vi "RFFE_Readback All Registers.vi"(8 "error out":errorcluster, 10 "RB All Regs":bool=TRUE, 11 "VISA IN":refnum<visa-resource-name>) -> (0 "error out 2":errorcluster, 2 "ALL Regs RB":string[](array[string]), 3 "VISA OUT":refnum<visa-resource-name>)   [LabVIEW 2017]
panel:
  out "Status":string="Idle....."
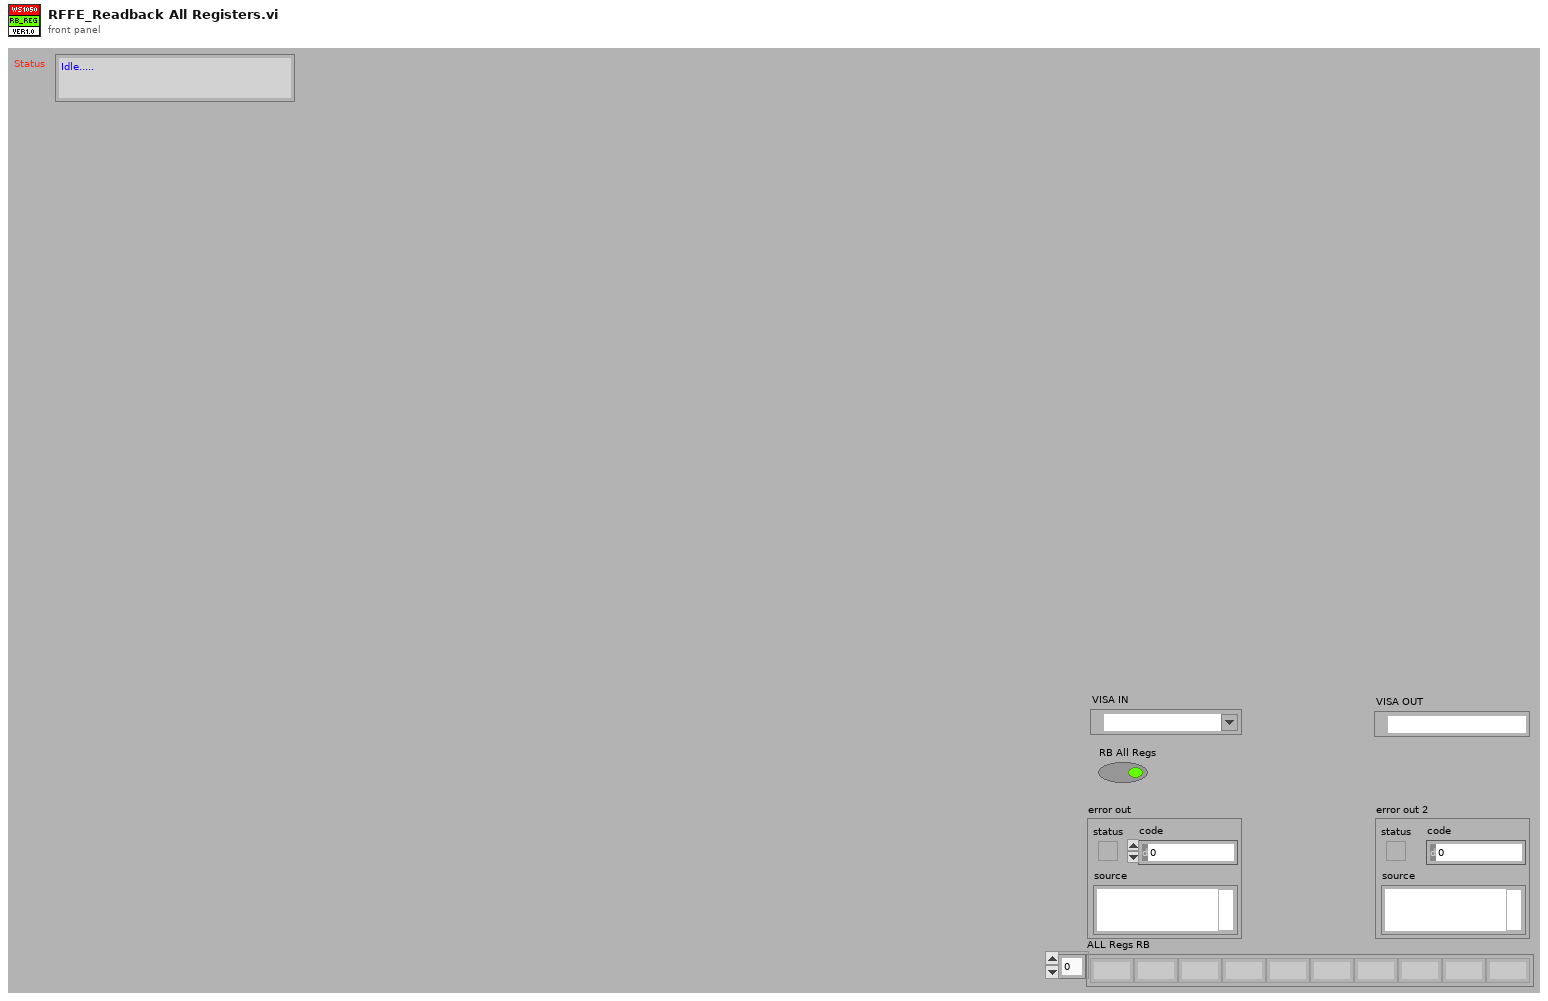
[diagram p1: front panel]
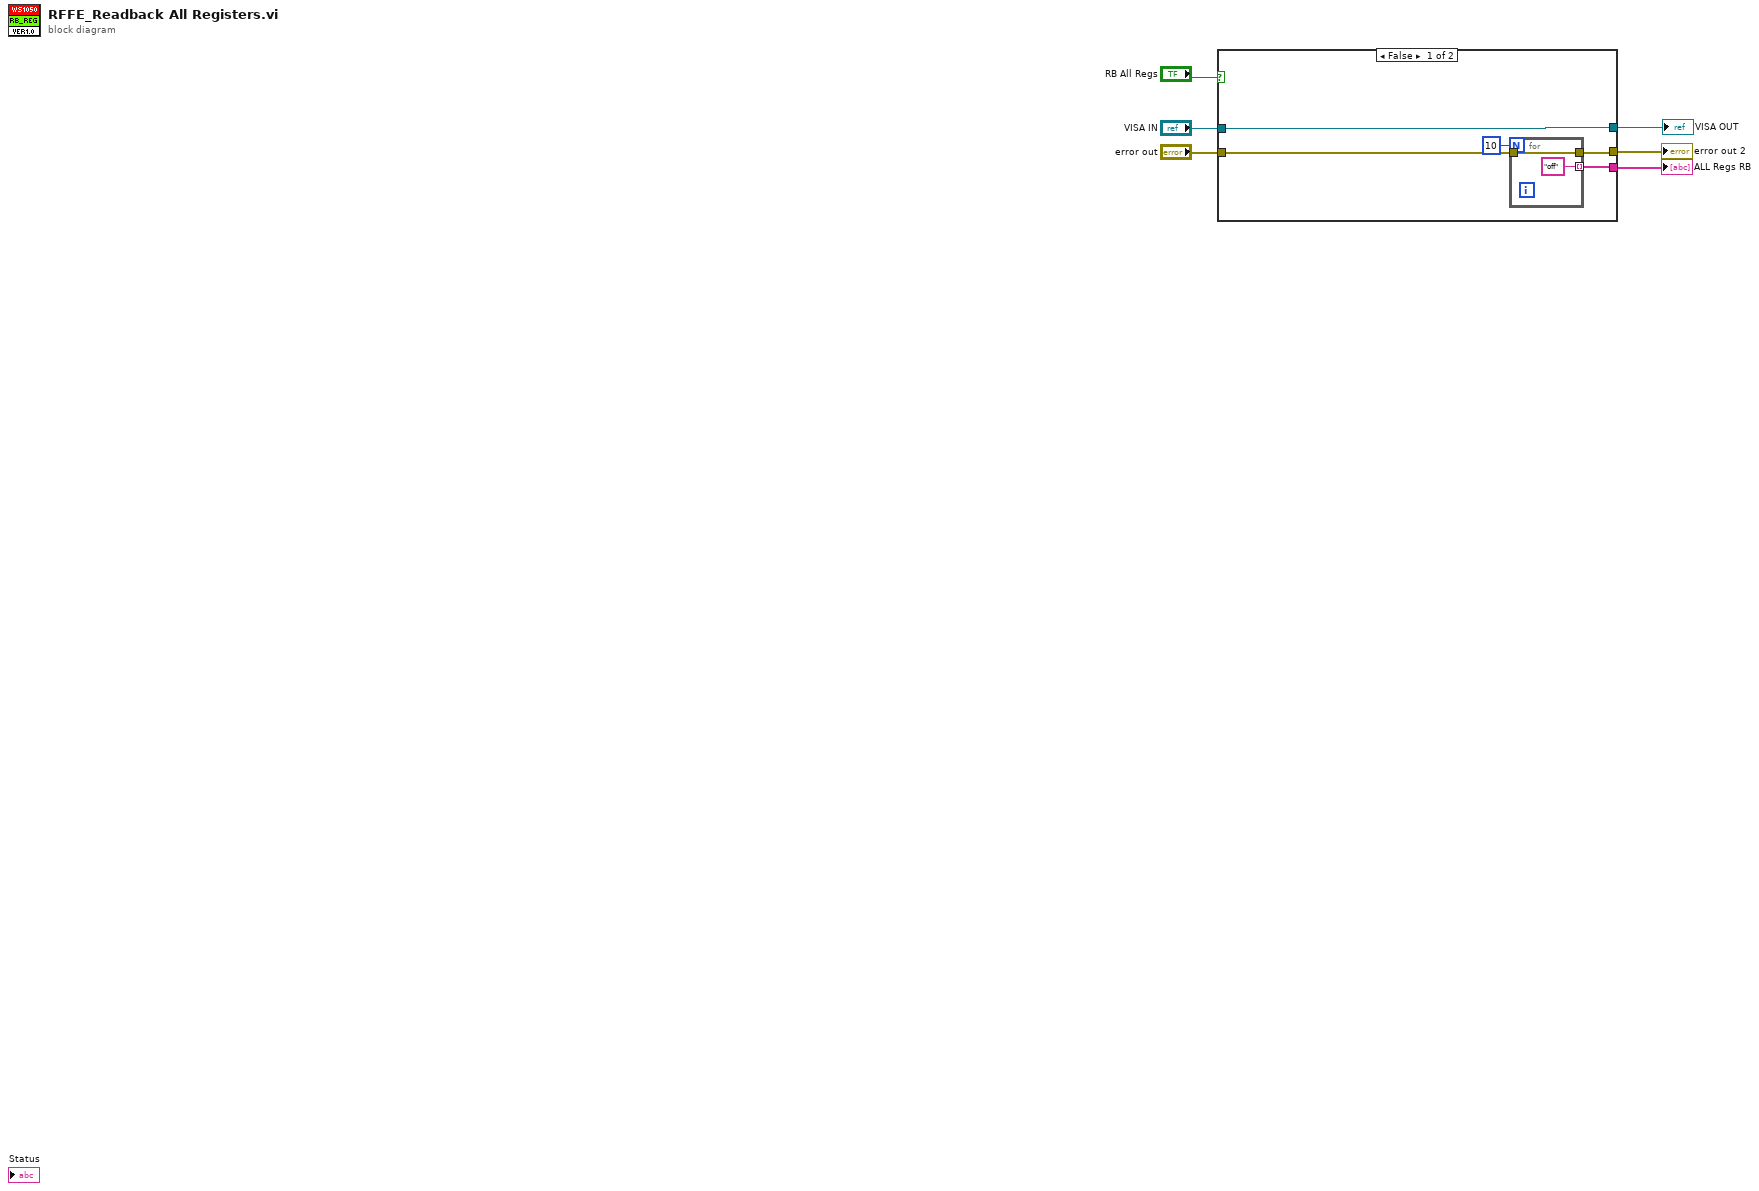
[diagram p0: block diagram]
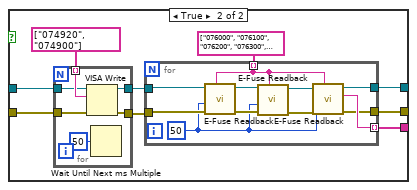
[diagram p2: hidden frame]
diagram:
  n1 = case shown="False" "RB All Regs" {
    tunnel: [w7 w21] -> w1
    tunnel: "error out" -> [w10 w16]
    tunnel: [w9 w19] -> w2
    tunnel: "VISA IN" -> [w11 w17]
    tunnel: [w11 w22] -> w4
    frame False {
      n2 = for {
        N: 10 -> [_]
        tunnel: w10 -> [w13]
        tunnel: [w13] -> w9
        tunnel: ["off"] -> w7 mode=indexing
      }
    }
    frame True {
      n3 = for {
        tunnel: w16 -> [w28]
        tunnel: string[] ["074920", "074900"] -> [w27] mode=indexing
        tunnel: w17 -> [w26]
        tunnel: [w24] -> w14
        tunnel: [w25] -> w15
        n4 = VISA Write(VISA resource name=w26, write buffer=w27, error in (no error)=w28) -> (VISA resource name out=w25:refnum<visa-resource-name>, error out=w24:errorcluster)  [unwired: 1 out]
        n5 = Wait Until Next ms Multiple(millisecond multiple=u32 50) -> ()  [unwired: 1 out]
      }
      n6 = for {
        tunnel: w14 -> [w33]
        tunnel: w15 -> [w32]
        tunnel: [w36] -> w22
        tunnel: [w37] -> w21 mode=indexing
        tunnel: string[] ["076000", "076100", "076200", "076300", "076400", "076500", "076600", "076700", "076800", "076900"] -> [w30] mode=indexing
        tunnel: [w35] -> w19
        w29 = u32 50 ("delay before read (ms)")
        n7 = call "E-Fuse Readback.vi"("write buffer"=w30, "error in (no error)"=w33, "delay before read (ms)"=w29, "VISA resource name"=w32) -> ("error out"=w34:errorcluster, "VISA resource name out"=w31:refnum<visa-resource-name>)  [unwired: 5 in, 1 out]
        n8 = call "E-Fuse Readback.vi"("write buffer"=w30, "error in (no error)"=w34, "delay before read (ms)"=w29, "VISA resource name"=w31) -> ("error out"=w38:errorcluster, "VISA resource name out"=w39:refnum<visa-resource-name>)  [unwired: 5 in, 1 out]
        n9 = call "E-Fuse Readback.vi"("write buffer"=w30, "error in (no error)"=w38, "delay before read (ms)"=w29, "VISA resource name"=w39) -> ("error out"=w35:errorcluster, "EFuse Read Back"=w37:string, "VISA resource name out"=w36:refnum<visa-resource-name>)  [unwired: 5 in]
      }
    }
  }
  "VISA OUT" <- w4
  "error out 2" <- w2
  "ALL Regs RB" <- w1
